vi "process-sync-start-test.vi"(8 "error in (no error)":errorcluster) -> (0 "error out":errorcluster)   [LabVIEW 2021]
uses:
  _test-support-SMOs/SMO.DynamicLauncher/SMO.DynamicLauncher.lvclass
  C:/Repositories/SMO/src/SMO/SMO.lvclass
  _test-support-SMOs/SMO.DynamicLauncher/SMO.DynamicLauncher.lvclass/SMO.DynamicLauncher.ctl
  <vilib>/addons/_JKI Toolkits/Caraya/classes/Assert/Assert Not Error.vi
  <vilib>/addons/_JKI Toolkits/Caraya/classes/Test/Test.lvclass
  src/SMO/SMO.lvclass
  <vilib>/addons/_JKI Toolkits/Caraya/classes/Assert/Assert.lvclass
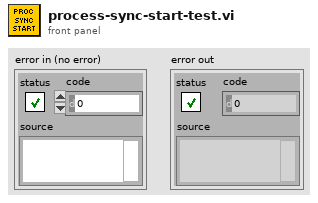
[diagram p1: front panel]
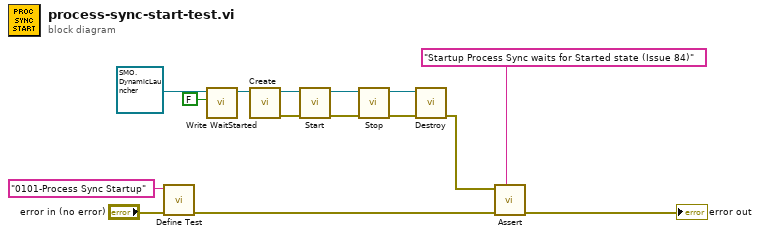
[diagram p0: block diagram]
diagram:
  n1 = call <vilib>:"Define Test.vi"("error in (no error)"="error in (no error)", "Label (VI Title)"="0101-Process Sync Startup") -> ("error out"=w6:errorcluster)  [unwired: 9 in]
  n2 = call "Write WaitStarted.vi"("WaitStarted"=FALSE, "SMO.DynamicLauncher in"=refnum<class "SMO.DynamicLauncher.lvclass"> refnum ("SMO.DynamicLauncher.lvclass")) -> ("SMO.DynamicLauncher out"=w2:refnum<class "SMO.DynamicLauncher.lvclass">)  [unwired: 9 in]
  n3 = call "Create.vi"("SMO"=w2) -> ("error out"=w13:errorcluster, "SMO out"=w14:refnum<class "SMO.DynamicLauncher.lvclass">)  [unwired: 8 in, 1 out]
  n4 = call "Start.vi"("error in (no error)"=w13, "SMO"=w14) -> ("error out"=w11:errorcluster, "SMO out"=w12:refnum<class "SMO.DynamicLauncher.lvclass">)  [unwired: 8 in]
  n5 = call "Stop.vi"("error in (no error)"=w11, "SMO"=w12) -> ("error out"=w10:errorcluster, "SMO out"=w9:refnum<class "SMO.DynamicLauncher.lvclass">)  [unwired: 8 in]
  n6 = call "Destroy.vi"("error in (no error)"=w10, "SMO"=w9) -> ("error out"=w7:errorcluster)  [unwired: 9 in]
  n7 = call-poly <vilib>:"Assert.vi"("Label"="Startup Process Sync waits for Started state (Issue 84)" ("Label (VI Title)"), "error in (no error)"=w6, "Not Error?"=w7) -> ("error out"=→"error out":errorcluster)  [unwired: 8 in]
